vi "Fast Item Rename FuncGlobal.vi"(5 "Action":enum16{"Open or Add", "Close Ref"}(ring), 8 "error in (no error)":errorcluster, 10 "New Name":string, 11 "Item Ref in":T1 format="%.0x") -> (0 "error out":errorcluster, 2 "Request invalid?":bool, 3 "Item Ref out":T1 format="%.0x")   [LabVIEW 2011]
doc: "Applies a <B>New Name</B> to the item specified by <B>Item Ref in</B>. If the <B>New Name</B> you specify already exists in the same section, this VI does nothing and the <B>Request invalid?</B> indicator returns TRUE."
uses:
  <vilib>/NI Veristand/Custom Device API/Custom Device Item Ref.ctl
  <vilib>/NI Veristand/Custom Device API/Custom Device API.lvlib
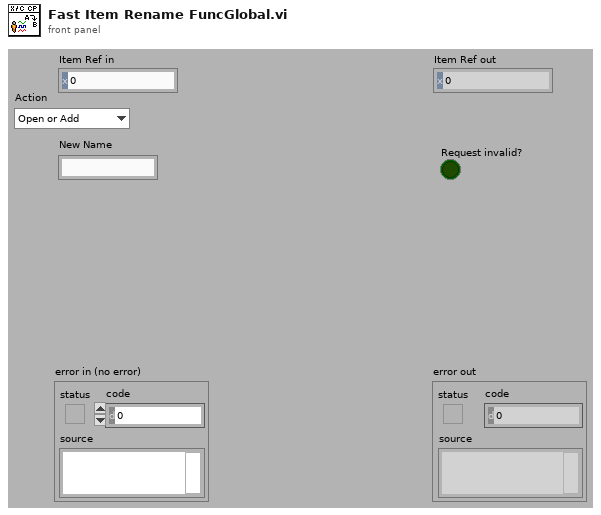
[diagram p1: front panel]
types:
  T1 = typedef "Custom Device API.lvlib/Custom Device Item Ref.ctl" = u64
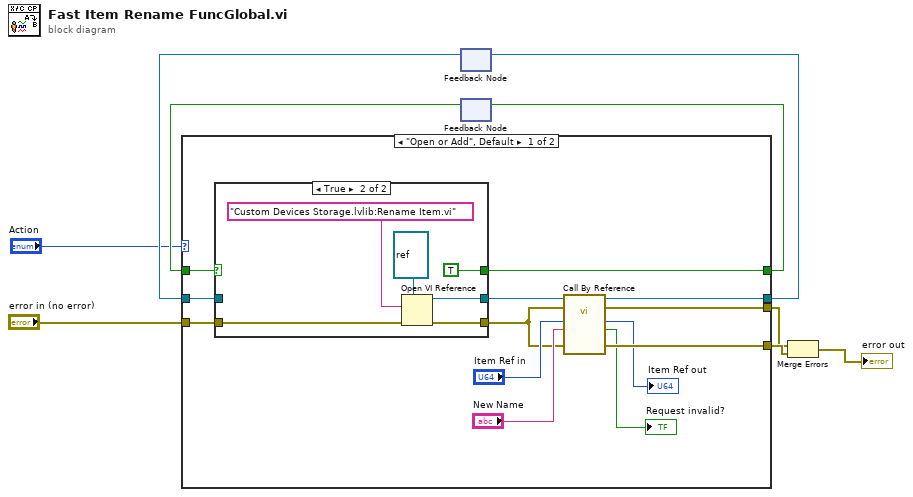
[diagram p0: block diagram]
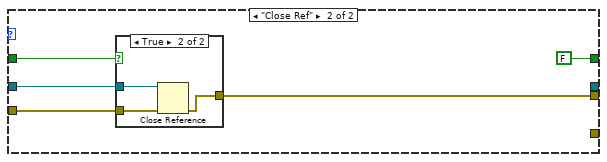
[diagram p3: hidden frame]
diagram:
  n1 = feedback #1() -> (w4:refnum<vi>)  [unwired: 1 in]
  n2 = feedback #2() -> (w2:bool)  [unwired: 1 in]
  n3 = case shown="\"Open or Add\", Default" "Action" {
    tunnel: [w22 _] -> w9
    tunnel: "error in (no error)" -> [w17 w36]
    tunnel: [w14 w33] -> w6
    tunnel: [w13 _] -> w5
    tunnel: w4 -> [w12 w35]
    tunnel: [w11 FALSE] -> w3
    tunnel: w2 -> [w10 w34]
    frame "Open or Add", Default {
      n4 = case shown="True" w10 {
        selector: w10 -> [w24 _]
        tunnel: w17 -> [w23 w29]
        tunnel: [w25 w28] -> w16
        tunnel: [w23 w27] -> w15
        tunnel: w12 -> [w25 _]
        tunnel: [w24 TRUE] -> w11
        frame False {
        }
        frame True {
          n5 = Open VI Reference(type specifier VI Refnum (for type only)=refnum<vi> refnum, vi path="Custom Devices Storage.lvlib:Rename Item.vi", error in (no error)=w29) -> (vi reference=w28:refnum<vi>, error out=w27:errorcluster)  [unwired: 3 out]
        }
      }
      n6 = call-by-ref "?"(reference=w16, error in=w15, 8:"error in (no error)"=w15, "New Name"="New Name", "Item Ref in"="Item Ref in") -> (reference out=w13:refnum<vi>, error out=w14:errorcluster, 0:"error out"=w22:errorcluster, "Request invalid?"=→"Request invalid?":bool, "Item Ref out"=→"Item Ref out":T1)  [unwired: 6 in]
    }
    frame "Close Ref" {
      n7 = case shown="True" w34 {
        tunnel: w36 -> [w37 w40]
        tunnel: w35 -> [_ w39]
        tunnel: [w37 w38] -> w33
        frame False {
        }
        frame True {
          n8 = Close Reference(reference=w39, error in (no error)=w40) -> (error out=w38:errorcluster)
        }
      }
    }
  }
  n9 = feedback-in #1(w5) -> ()
  n10 = feedback-in #2(w3) -> ()
  n11 = Merge Errors(w6, w9) -> (→"error out":errorcluster)
